vi "QKD-BB84.vi"() -> ()   [LabVIEW 2020]
uses:
  QuSim/QuVI_Wire (initial).vi
  Gates/Polymorphs/Pauli-X_s.vi
  Analysis/Inspect VIs/Bloch Sphere - Display.vi
panel:
  out "Shots":i32=100
  out "Sifted Key Size":i32
  out "Bob's Sifted Key":bool[](array[boolean])
  out "Alice's Sifted Key":bool[](array[boolean])
  out "QBER Meter":dbl(knob) scale=0.0..100.0
  in  "Eavesdropper":bool
  # "BB84 Quantum Key Distribution"
  # "This simulation demonstrates how quantum mechanics guarantees communication security. \n- Run the VI to generate a shared key.\n- Toggle the Eavesdropper to observe how the laws of physics prevent undetected interception."
  # "Eavesdropper (Eve) Presence\nOFF: The quantum channel is secure. Photons travel undisturbed from Alice to Bob.\nON: Eve intercepts the transmission! She measures the photons mid-flight (collapsing their quantum state) and sends forged replacements to Bob, breaking the quantum correlation."
  # "The Sifted Keys (Shared Secret)\nThese arrays display the final key after the \"Sifting\" phase over a public channel. Alice and Bob have discarded any bits where they randomly chose different measurement bases.\nSecure Channel: Alice and Bob's arrays will match perfectly.\nCompromised Channel: Errors will appear between the two arrays due to Eve's interference."
  # "This meter calculates the percentage of mismatched bits between Alice and Bob's sifted keys.\n 0%: Cryptographically secure.\n~25%: Eavesdropper detected! Eve's forced measurements inevitably scramble the quantum states, leaving a permanent mathematical footprint."
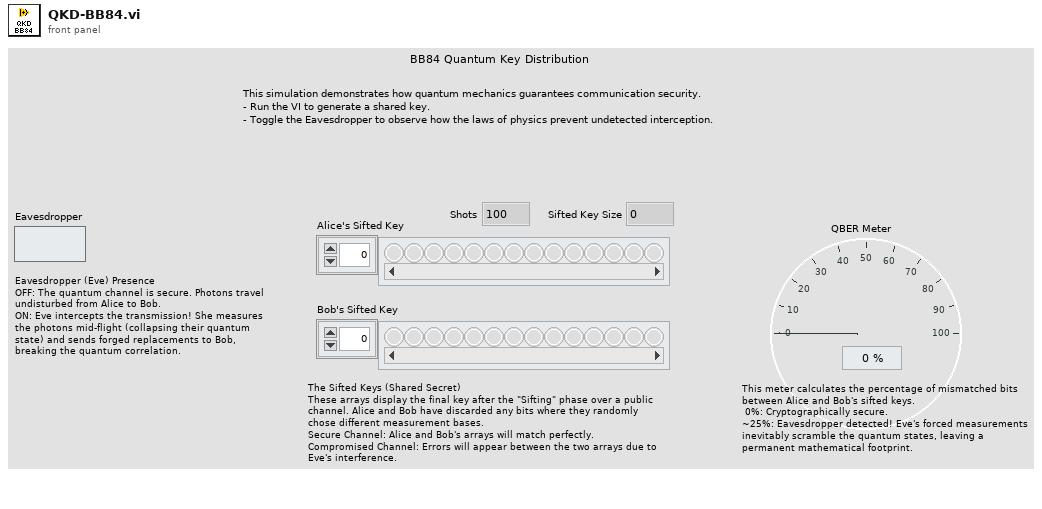
[diagram p1: front panel]
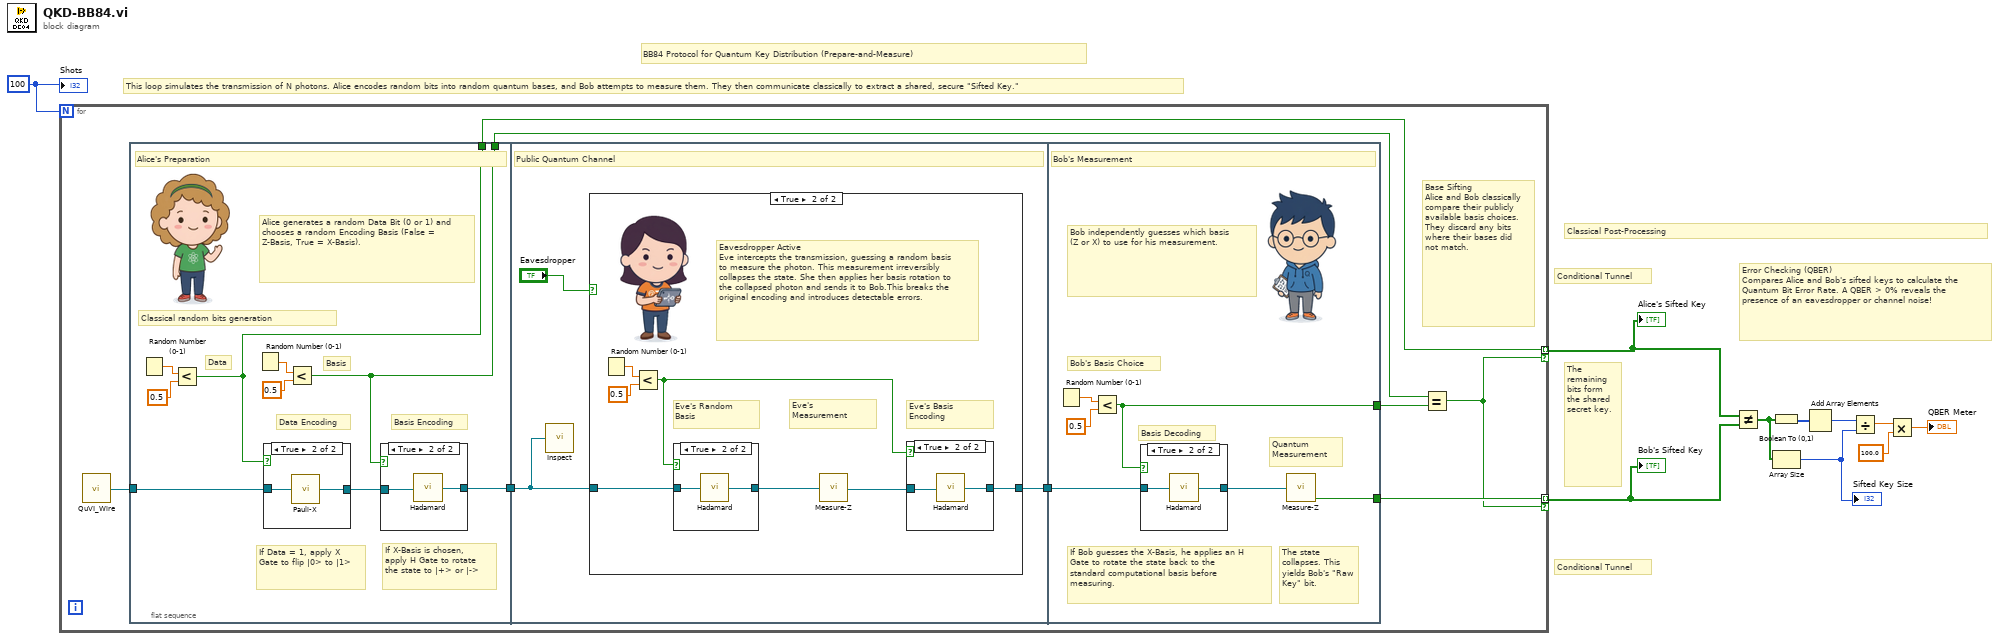
[diagram p0: block diagram]
diagram:
  w10 = 100
  # "Conditional Tunnel"
  # "Error Checking (QBER)\nCompares Alice and Bob's sifted keys to calculate the Quantum Bit Error Rate. A QBER > 0% reveals the presence of an eavesdropper or channel noise!"
  # "The remaining bits form the shared secret key."
  # "Conditional Tunnel"
  # "This loop simulates the transmission of N photons. Alice encodes random bits into random quantum bases, and Bob attempts to measure them. They then communicate classically to extract a shared, secure \"Sifted Key.\""
  # "BB84 Protocol for Quantum Key Distribution (Prepare-and-Measure)"
  # "Classical Post-Processing"
  n1 = for {
    N: w10 -> [_]
    tunnel: [w15] -> w1 mode=indexing if=w11
    tunnel: [w14] -> w2 mode=indexing if=w11
    # "Base Sifting \nAlice and Bob classically compare their publicly available basis choices. They discard any bits where their bases did not match."
    n2 = call-poly "QuVI_Wire.vi"() -> ("QuWire out"=w16:refnum<class "QuWire.lvclass">)  [unwired: 14 in, 1 out]
    n3 = flat-sequence {
      tunnel: w16 -> [w25]
      tunnel: [w21] -> w18
      tunnel: [w20] -> w14
      tunnel: [w19] -> w13
      tunnel: w18 -> [w34]
      tunnel: [w36] -> w17
      tunnel: w17 -> [w54]
      tunnel: [w52] -> w12
      tunnel: [w51] -> w15
      frame #0 {
        # "Basis"
        # "Data"
        # "If X-Basis is chosen, apply H Gate to rotate the state to |+> or |->"
        # "If Data = 1, apply X Gate to flip |0> to |1>"
        # "Alice generates a random Data Bit (0 or 1) and chooses a random Encoding Basis (False = Z-Basis, True = X-Basis)."
        # "Classical random bits generation"
        # "Basis Encoding"
        # "Data Encoding"
        # "Alice's Preparation"
        n4 = Random Number (0-1)() -> (number: 0 to 1=w27:dbl)
        n5 = Less?(x=w27, y=0.5 ("x")) -> (x < y?=w20:bool)
        n6 = Random Number (0-1)() -> (number: 0 to 1=w22:dbl)
        n7 = case shown="True" w20 {
          tunnel: w25 -> [w28 w30]
          tunnel: [w28 w29] -> w24
          frame False {
          }
          frame True {
            n8 = call-poly "Pauli-X.vi"("QuWire in"=w30) -> ("QuWire out"=w29:refnum<class "QuWire.lvclass">)  [unwired: 14 in]
          }
        }
        n9 = Less?(x=w22, y=0.5 ("x")) -> (x < y?=w19:bool)
        n10 = case shown="True" w19 {
          tunnel: w24 -> [w31 w33]
          tunnel: [w31 w32] -> w21
          frame False {
          }
          frame True {
            n11 = call "Hadamard.vi"("QuWire in"=w33) -> ("QuWire out"=w32:refnum<class "QuWire.lvclass">)  [unwired: 14 in]
          }
        }
      }
      frame #1 {
        # "Public Quantum Channel"
        n12 = call-poly "Inspect.vi"("QuWire in"=w34) -> ()  [unwired: 15 in]
        n13 = case shown="True" "Eavesdropper" {
          tunnel: w34 -> [w37 w44]
          tunnel: [w37 w42] -> w36
          frame False {
          }
          frame True {
            # "Eve's Basis Encoding"
            # "Eve's Measurement"
            # "Eve's Random Basis"
            # "Eavesdropper Active\nEve intercepts the transmission, guessing a random basis to measure the photon. This measurement irreversibly collapses the state. She then applies her basis rotation to the collapsed photon and sends it to Bob.This breaks the original encoding and introduces detectable errors."
            n14 = Random Number (0-1)() -> (number: 0 to 1=w41:dbl)
            n15 = Less?(x=w41, y=0.5 ("x")) -> (x < y?=w43:bool)
            n16 = case shown="True" w43 {
              tunnel: w44 -> [w45 w47]
              tunnel: [w45 w46] -> w39
              frame False {
              }
              frame True {
                n17 = call "Hadamard.vi"("QuWire in"=w47) -> ("QuWire out"=w46:refnum<class "QuWire.lvclass">)  [unwired: 14 in]
              }
            }
            n18 = call "Measure-Z.vi"("QuWire in"=w39) -> ("QuWire out"=w38:refnum<class "QuWire.lvclass">)  [unwired: 13 in, 1 out]
            n19 = case shown="True" w43 {
              tunnel: w38 -> [w48 w50]
              tunnel: [w48 w49] -> w42
              frame False {
              }
              frame True {
                n20 = call "Hadamard.vi"("QuWire in"=w50) -> ("QuWire out"=w49:refnum<class "QuWire.lvclass">)  [unwired: 14 in]
              }
            }
          }
        }
      }
      frame #2 {
        # "If Bob guesses the X-Basis, he applies an H Gate to rotate the state back to the standard computational basis before measuring."
        # "The state collapses. This yields Bob's \"Raw Key\" bit."
        # "Quantum Measurement"
        # "Bob independently guesses which basis (Z or X) to use for his measurement."
        # "Bob's Basis Choice"
        # "Basis Decoding"
        # "Bob's Measurement"
        n21 = Random Number (0-1)() -> (number: 0 to 1=w56:dbl)
        n22 = Less?(x=w56, y=0.5 ("x")) -> (x < y?=w52:bool)
        n23 = case shown="True" w52 {
          tunnel: w54 -> [w57 w59]
          tunnel: [w57 w58] -> w53
          frame False {
          }
          frame True {
            n24 = call "Hadamard.vi"("QuWire in"=w59) -> ("QuWire out"=w58:refnum<class "QuWire.lvclass">)  [unwired: 14 in]
          }
        }
        n25 = call "Measure-Z.vi"("QuWire in"=w53) -> ("Classical bit"=w51:bool)  [unwired: 13 in, 1 out]
      }
    }
    n26 = Equal?(x=w13, y=w12) -> (x = y?=w11:bool)
  }
  "Alice's Sifted Key" <- w2
  "Bob's Sifted Key" <- w1
  n27 = Not Equal?(x=w2, y=w1) -> (x != y?=w3:bool[])
  n28 = Boolean To (0,1)(Boolean=w3) -> (0, 1=w9:i16[])
  n29 = Array Size(array=w3) -> (size(s)=w7:i32)
  "Sifted Key Size" <- w7
  n30 = Add Array Elements(numeric array=w9) -> (sum=w8:i16)
  n31 = Divide(x=w8, y=w7) -> (x/y=w6:dbl)
  n32 = Multiply(x=w6, y=100.0) -> (x*y=→"QBER Meter":dbl)
  "Shots" <- w10
